vi "readVariable_I32.vi"(8 "error in (no error)":errorcluster, 10 "URL":string, 11 "Client In":refnum<class "Client.lvclass">) -> (0 "error out":errorcluster, 1 "val":i32, 2 "return type":i32, 3 "Client out":refnum<class "Client.lvclass">)   [LabVIEW 2017, in "opcua.lvlib" / "Client.lvclass"]
uses:
  Client.lvclass
  Client.lvclass/Client.ctl
  opcua32.dll
  opcua.lvlib
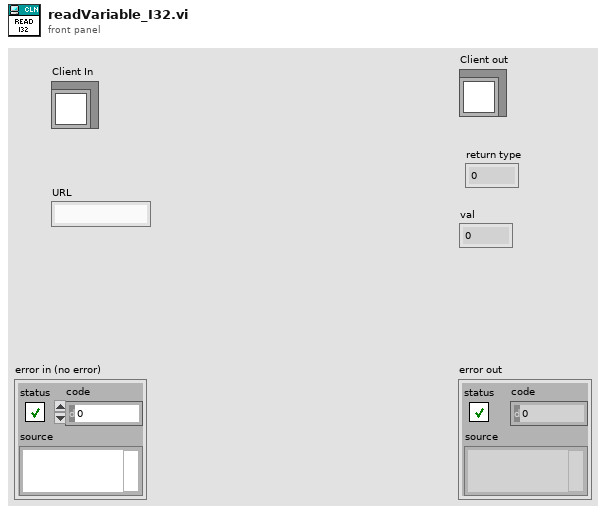
[diagram p1: front panel]
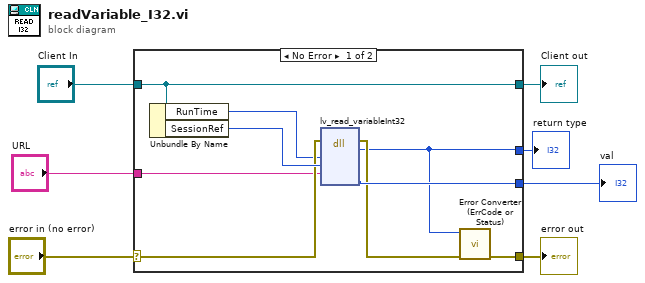
[diagram p0: block diagram]
diagram:
  n1 = case shown="No Error" "error in (no error)" {
    selector: "error in (no error)" -> [w15 w17]
    tunnel: [w9 w17] -> w6
    tunnel: [w14 w18] -> w5
    tunnel: "Client In" -> [w14 w18]
    tunnel: "URL" -> [w12 _]
    tunnel: [w8 _] -> w2
    tunnel: [w11 _] -> w1
    frame No Error {
      n2 = Unbundle By Name(w14) -> ("RunTime"=w13:u64, "SessionRef"=w16:u64)
      n3 = dll-call lib="C:/Users/Andrey/Desktop/opcua-labview/opcua-lvlib/opcua*.dll" fn="lv_read_variableInt32"(error in=w15, "runtime"=w13, "client_ref"=w16, "var"=w12) -> (error out=w10:errorcluster, "return type"=w8:i32, "val"=w11:i32)  [unwired: 6 in, 1 out]
      n4 = call "Error Converter (ErrCode or Status).vi"("error in (no error)"=w10, "error code"=w8) -> ("error out"=w9:errorcluster)  [unwired: 9 in]
    }
    frame Error {
    }
  }
  "error out" <- w6
  "Client out" <- w5
  "return type" <- w2
  "val" <- w1
